vi "init alias tree.vi"(8 "error in (no error)":errorcluster, 9 "allow multi-select":bool, 10 "show checkbox":bool, 11 "alias-tree in":refnum<class "alias-tree.lvclass">) -> (0 "error out":errorcluster, 3 "alias-tree out":refnum<class "alias-tree.lvclass">)   [LabVIEW 2017, in "vs-tree-utility.lvlib" / "alias-tree.lvclass"]
uses:
  alias-tree.lvclass
  NationalInstruments.VeriStand.SystemStorageUI
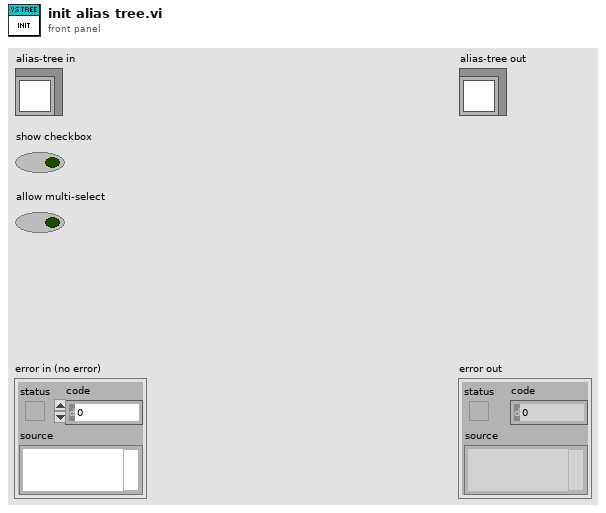
[diagram p1: front panel]
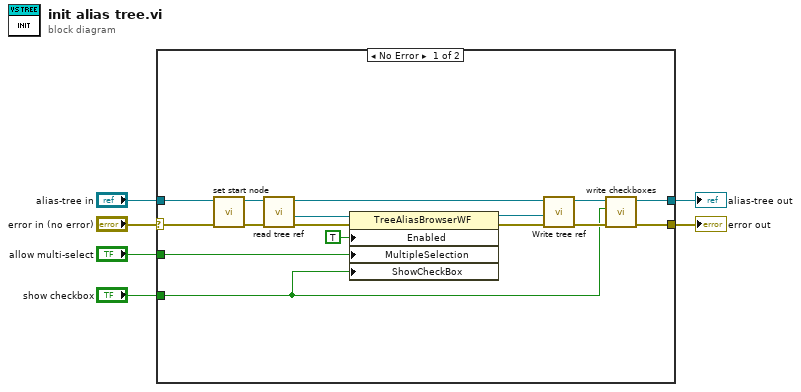
[diagram p0: block diagram]
diagram:
  n1 = case shown="No Error" "error in (no error)" {
    selector: "error in (no error)" -> [w20 w24]
    tunnel: [w10 w24] -> w5
    tunnel: [w8 w23] -> w3
    tunnel: "alias-tree in" -> [w18 w23]
    tunnel: "show checkbox" -> [w7 _]
    tunnel: "allow multi-select" -> [w21 _]
    frame No Error {
      n2 = call-dynamic "set start node.vi"("error in (no error)"=w20, "alias-tree in"=w18) -> ("error out"=w19:errorcluster, "alias-tree out"=w15:refnum<class "alias-tree.lvclass">)  [unwired: 8 in]
      n3 = call-dynamic "read tree ref.vi"("error in (no error)"=w19, "alias-tree in"=w15) -> ("error out"=w16:errorcluster, "tree ref"=w14:refnum<k24>, "alias-tree out"=w11:refnum<class "alias-tree.lvclass">)  [unwired: 7 in]
      n4 = property class="TreeAliasBrowserWF"(reference=w14, error in=w16, "Enabled"=TRUE, "MultipleSelection"=w21, "ShowCheckBox"=w7) -> (reference out=w12:refnum<k24>, error out=w17:errorcluster)
      n5 = call-dynamic "Write tree ref.vi"("error in (no error)"=w17, "tree ref"=w12, "alias-tree in"=w11) -> ("error out"=w13:errorcluster, "alias-tree out"=w9:refnum<class "alias-tree.lvclass">)  [unwired: 7 in]
      n6 = call-dynamic "write checkboxes.vi"("error in (no error)"=w13, "checkboxes"=w7, "alias-tree in"=w9) -> ("error out"=w10:errorcluster, "alias-tree out"=w8:refnum<class "alias-tree.lvclass">)  [unwired: 7 in]
    }
    frame Error {
    }
  }
  "error out" <- w5
  "alias-tree out" <- w3
